vi "roboRIO v1.0 Read DIO.vi"(8 "error in (no error)":errorcluster, 10 "Channel List":T3, 11 "myRIO Ref In":T1) -> (0 "error out":errorcluster, 2 "bool Value List":bool[](array[boolean]), 3 "myRIO Ref Out":T1)   [LabVIEW 2021]
uses:
  <vilib>/myRIO/Common/Instrument Driver Framework/myRIO v1.0/DIO/typedefs/DIO Channels List.ctl
  <vilib>/myRIO/Common/Instrument Driver Framework/myRIO v1.0/DIO/typedefs/DIO Channels Enum.ctl
  <vilib>/myRIO/Common/Instrument Driver Framework/Utilities/typedefs/myRIO v1.0 Reference.ctl
  <vilib>/myRIO/Common/Instrument Driver Framework/Utilities/typedefs/Generic FPGA Reference.ctl
  <vilib>/myRIO/Common/Instrument Driver Framework/roboRIO v1.0/DIO/typedefs/roboRIO DIO FPGA Reference.ctl
  <vilib>/myRIO/Common/Instrument Driver Framework/roboRIO v1.0/DIO/typedefs/roboRIO DIO Bank Enum.ctl
  <vilib>/Utility/error.llb/Error Cluster From Error Code.vi
  <vilib>/rvi/errors/niLvFpgaAdjustHostInterfaceError.vi
  <vilib>/rvi/interface/nirviReadWriteControl/nirviReadWriteControl.xnode
  <vilib>/rvi/interface/Simulation/niFpgaSimulationCallBeginRW.vi
  NiFpgaLv.dll
panel:
  # "This VI reads boolean values from a list of user specified channels on\nthe myRIO v1.0 hardware. The value is read on the FPGA as a bit and \nconverted to a boolean. Please see Block Diagram for details."
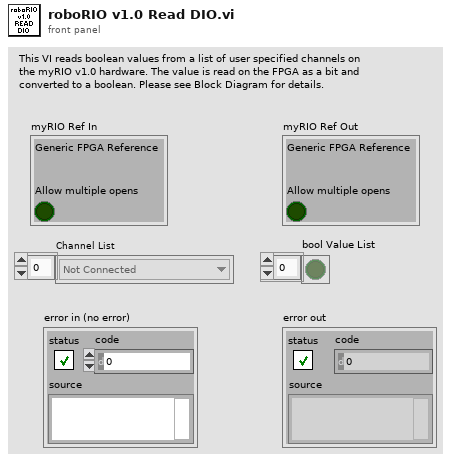
[diagram p1: front panel]
types:
  T1 = typedef "myRIO v1.0 Reference.ctl" = cluster{"Generic FPGA Reference":T2, "Allow multiple opens":bool}
  T2 = typedef "Generic FPGA Reference.ctl" = refnum<k20>
  T3 = typedef "DIO Channels List.ctl" = T4[]
  T4 = typedef "DIO Channels Enum.ctl" = enum16{"Not Connected", "C/DIO0", "C/DIO1", "C/DIO2", "C/DIO3", "C/DIO4", "C/DIO5", "C/DIO6", "C/DIO7", "A/DIO0", "A/DIO1", "A/DIO2", "A/DIO3", "A/DIO4", "A/DIO5", "A/DIO6", "A/DIO7", "A/DIO8", "A/DIO9", "A/DIO10", "A/DIO11", "A/DIO12", "A/DIO13", "A/DIO14", "A/DIO15", "A/DIO16", "A/DIO17", "A/DIO18", "A/DIO19", "B/DIO0", "B/DIO1", "B/DIO2", "B/DIO3", "B/DIO4", "B/DIO5", "B/DIO6", "B/DIO7", "B/DIO8", "B/DIO9", "B/DIO10", "B/DIO11", "B/DIO12", "B/DIO13", "B/DIO14", "B/DIO15", "B/DIO16", "B/DIO17", "B/DIO18", "B/DIO19", "LED0", "LED1", "LED2", "LED3", "Button0", "DIO/DIO0", "DIO/DIO1", "DIO/DIO2", "DIO/DIO3", "DIO/DIO4", "DIO/DIO5", "DIO/DIO6", "DIO/DIO7", "DIO/DIO8", "DIO/DIO9", "SPI/CS0", "SPI/CS1", "SPI/CS2", "SPI/CS3", "LED RADIO (Green)", "LED RADIO (Red)", "LED COMM (Green)", "LED COMM (Red)", "LED MODE (Green)", "LED MODE (Red)"}
  T5 = typedef "roboRIO DIO Bank Enum.ctl" = enum32{"None", "B/DIO7:0", "B/DIO15:8", "DIO/DIO7:0", "DIO/DIO9:8", "SPI/CS3:0", "LED", "Button0"}
  T6 = typedef "roboRIO DIO FPGA Reference.ctl" = refnum<k20>
  T7 = typedef "roboRIO DIO Bitmask to Channel Map.ctl" = cluster{"DIO Bank Enum":T5, "Bit":i32}
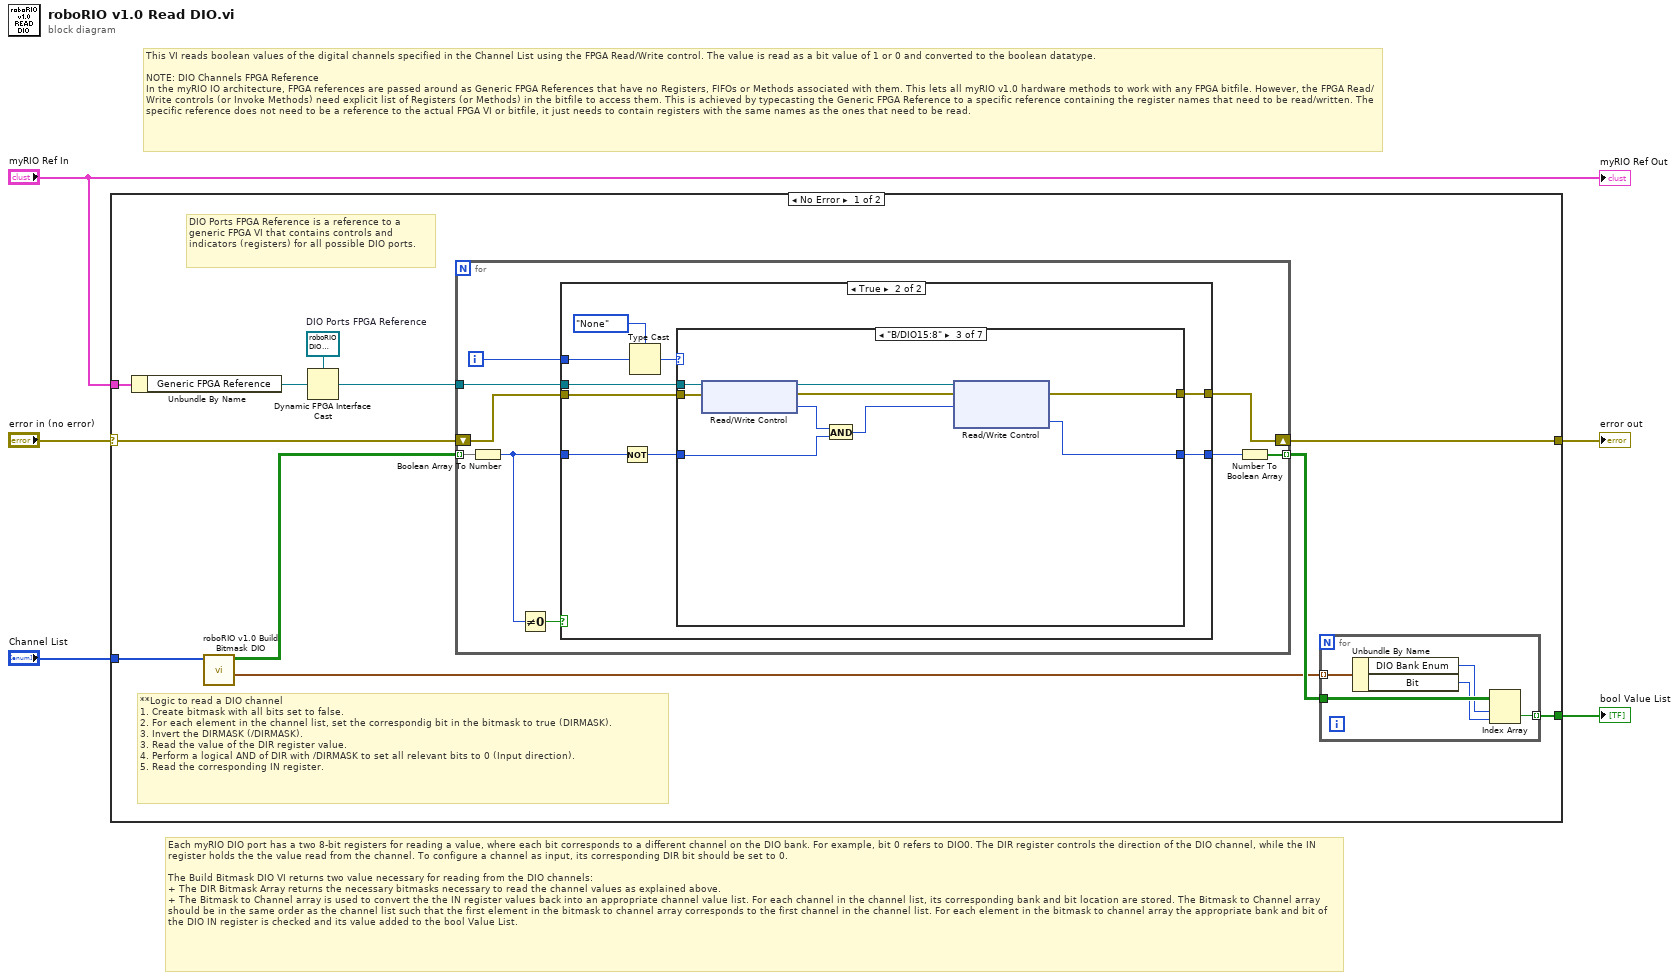
[diagram p0: block diagram]
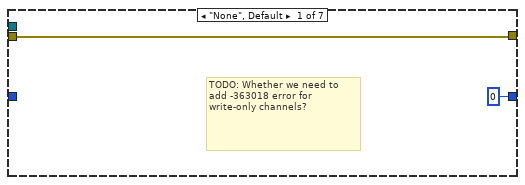
[diagram p3: hidden frame]
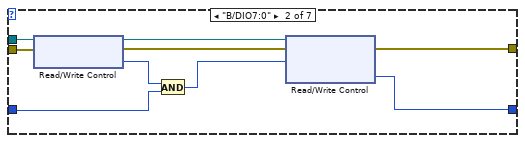
[diagram p4: hidden frame]
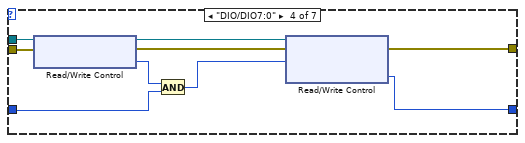
[diagram p5: hidden frame]
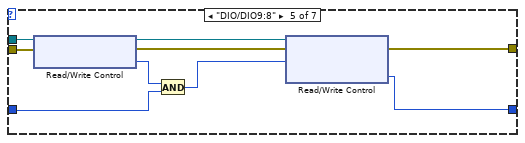
[diagram p6: hidden frame]
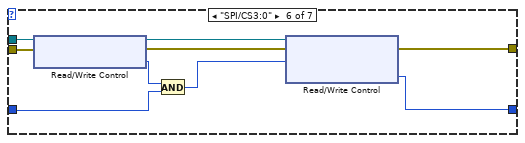
[diagram p7: hidden frame]
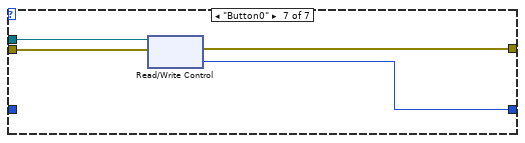
[diagram p8: hidden frame]
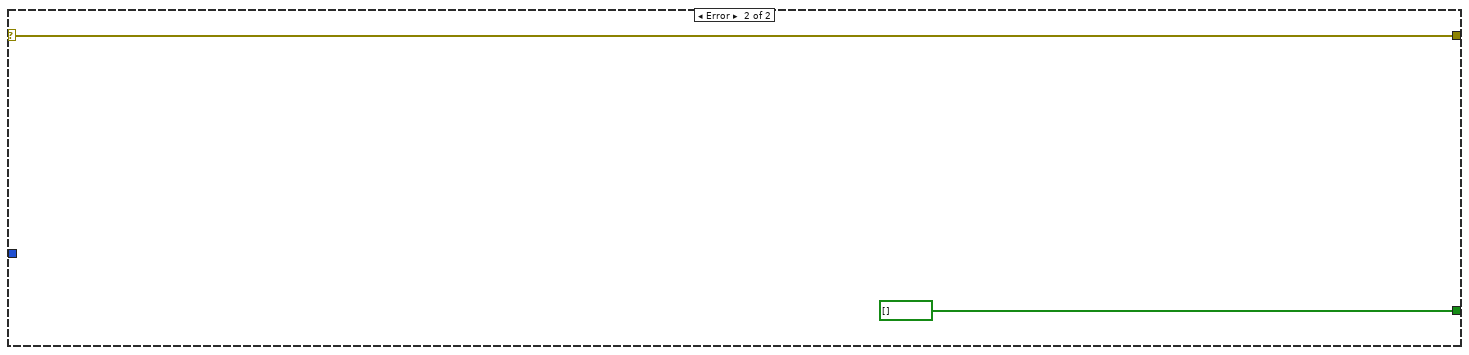
[diagram p9: hidden frame]
diagram:
  # "Each myRIO DIO port has a two 8-bit registers for reading a value, where each bit corresponds to a different channel on the DIO bank. For example, bit 0 refers to DIO0. The DIR register controls the direction of the DIO channel, while the IN register holds the the value read from the channel. To configure a channel as input, its corresponding DIR bit should be set to 0.\n\nThe Build Bitmask DIO VI returns two value necessary for reading from the DIO channels:\n+ The DIR Bitmask Array returns the necessary bitmasks necessary to read the channel values as explained above. \n+ The Bitmask to Channel array is used to convert the the IN register values back into an appropriate channel value list. For each channel in the channel list, its corresponding bank and bit location are stored. The Bitmask to Channel array should be in the same order as the channel list such that the first element in the bitmask to channel array corresponds to the first channel in the channel list. For each element in the bitmask to channel array the appropriate bank and bit of the DIO IN register is checked and its value added to the bool Value List."
  # "This VI reads boolean values of the digital channels specified in the Channel List using the FPGA Read/Write control. The value is read as a bit value of 1 or 0 and converted to the boolean datatype. \n\nNOTE: DIO Channels FPGA Reference\nIn the myRIO IO architecture, FPGA references are passed around as Generic FPGA References that have no Registers, FIFOs or Methods associated with them. This lets all myRIO v1.0 hardware methods to work with any FPGA bitfile. However, the FPGA Read/Write controls (or Invoke Methods) need explicit list of Registers (or Methods) in the bitfile to access them. This is achieved by typecasting the Generic FPGA Reference to a specific reference containing the register names that need to be read/written. The specific reference does not need to be a reference to the actual FPGA VI or bitfile, it just needs to contain registers with the same names as the ones that need to be read."
  n1 = case shown="No Error" "error in (no error)" {
    selector: "error in (no error)" -> [w7 w94]
    tunnel: "myRIO Ref In" -> [w13 _]
    tunnel: [w12 w94] -> w4
    tunnel: [w11 bool[] []] -> w2
    tunnel: "Channel List" -> [w10 _]
    frame No Error {
      w16 = T6 refnum  # DIO Ports FPGA Reference
      # "DIO Ports FPGA Reference is a reference to a generic FPGA VI that contains controls and indicators (registers) for all possible DIO ports."
      # "**Logic to read a DIO channel\n1. Create bitmask with all bits set to false.\n2. For each element in the channel list, set the correspondig bit in the bitmask to true (DIRMASK).\n3. Invert the DIRMASK (/DIRMASK).\n3. Read the value of the DIR register value.\n4. Perform a logical AND of DIR with /DIRMASK to set all relevant bits to 0 (Input direction).\n5. Read the corresponding IN register."
      n2 = Unbundle By Name(w13) -> ("Generic FPGA Reference"=w6:T2)
      n3 = call <vilib>:"roboRIO v1.0 Build Bitmask DIO.vi"("Channel List"=w10) -> ("Bitmask to Channel Array"=w8:T7[], "DIR Bitmask Array"=w9:bool[][])  [unwired: 8 in, 1 out]
      n4 = Dynamic FPGA Interface Cast(Session In=w16, Type=w6) -> (Session Out=w15:T6)
      n5 = for {
        tunnel: w9 -> [w28] mode=indexing
        tunnel: w15 -> [w30]
        shift-right: [w27] -> w12
        shift-left: w7 -> [w26]
        tunnel: [w24] -> w14 mode=indexing
        i -> [w29]
        n6 = Boolean Array To Number(Boolean array=w28) -> (number=w22:u8)
        n7 = Not Equal To 0?(x=w22) -> (x != 0?=w23:bool)
        n8 = case shown="True" w23 {
          tunnel: w30 -> [_ w41]
          tunnel: w29 -> [_ w40]
          tunnel: w22 -> [w31 w37]
          tunnel: [w32 w35] -> w27
          tunnel: w26 -> [w32 w34]
          tunnel: [w31 w33] -> w25
          frame False {
          }
          frame True {
            n9 = Not(x=w37) -> (.not. x?=w36:u8)
            n10 = Type Cast(type=roboRIO_DIO_Bank_Enum."None" ("DIO Bank Enum"), x=w40) -> (*(type *) &x=w38:T5)
            n11 = case shown="\"B/DIO15:8\"" w38 {
              tunnel: w41 -> [_ w52 w61 w70 w79 w88 w92]
              tunnel: w36 -> [_ w48 w57 w66 w75 w84 _]
              tunnel: [w43 w46 w55 w64 w73 w82 w91] -> w35
              tunnel: w34 -> [w43 w45 w54 w63 w72 w81 w90]
              tunnel: [u8 0 ("DIO.A_15:8.IN") w44 w53 w62 w71 w80 w89] -> w33
              frame "None", Default {
                # "TODO: Whether we need to add -363018 error for write-only channels?"
              }
              frame "B/DIO7:0" {
                n12 = xnode "Read/Write Control"("FPGA VI Reference In"=w52, "error in"=w45) -> ("FPGA VI Reference Out"=w51:T6, "error out"=w47:errorcluster, "DIO.B_7:0.DIR"=w50:u8)
                n13 = And(x=w50, y=w48) -> (x .and. y?=w49:u8)
                n14 = xnode "Read/Write Control"("FPGA VI Reference In"=w51, "error in"=w47, "DIO.B_7:0.DIR"=w49) -> ("error out"=w46:errorcluster, "DIO.B_7:0.IN"=w44:u8)  [unwired: 1 out]
              }
              frame "B/DIO15:8" {
                n15 = xnode "Read/Write Control"("FPGA VI Reference In"=w61, "error in"=w54) -> ("FPGA VI Reference Out"=w60:T6, "error out"=w56:errorcluster, "DIO.B_15:8.DIR"=w59:u8)
                n16 = And(x=w59, y=w57) -> (x .and. y?=w58:u8)
                n17 = xnode "Read/Write Control"("FPGA VI Reference In"=w60, "error in"=w56, "DIO.B_15:8.DIR"=w58) -> ("error out"=w55:errorcluster, "DIO.B_15:8.IN"=w53:u8)  [unwired: 1 out]
              }
              frame "DIO/DIO7:0" {
                n18 = xnode "Read/Write Control"("FPGA VI Reference In"=w70, "error in"=w63) -> ("FPGA VI Reference Out"=w69:T6, "error out"=w65:errorcluster, "DIO.DIO_7:0.DIR"=w68:u8)
                n19 = And(x=w68, y=w66) -> (x .and. y?=w67:u8)
                n20 = xnode "Read/Write Control"("FPGA VI Reference In"=w69, "error in"=w65, "DIO.DIO_7:0.DIR"=w67) -> ("error out"=w64:errorcluster, "DIO.DIO_7:0.IN"=w62:u8)  [unwired: 1 out]
              }
              frame "DIO/DIO9:8" {
                n21 = xnode "Read/Write Control"("FPGA VI Reference In"=w79, "error in"=w72) -> ("FPGA VI Reference Out"=w78:T6, "error out"=w74:errorcluster, "DIO.DIO_9:8.DIR"=w77:u8)
                n22 = And(x=w77, y=w75) -> (x .and. y?=w76:u8)
                n23 = xnode "Read/Write Control"("FPGA VI Reference In"=w78, "error in"=w74, "DIO.DIO_9:8.DIR"=w76) -> ("error out"=w73:errorcluster, "DIO.DIO_9:8.IN"=w71:u8)  [unwired: 1 out]
              }
              frame "SPI/CS3:0" {
                n24 = xnode "Read/Write Control"("FPGA VI Reference In"=w88, "error in"=w81) -> ("FPGA VI Reference Out"=w87:T6, "error out"=w83:errorcluster, "DIO.SPI_CS3:0.DIR"=w86:u8)
                n25 = And(x=w86, y=w84) -> (x .and. y?=w85:u8)
                n26 = xnode "Read/Write Control"("FPGA VI Reference In"=w87, "error in"=w83, "DIO.SPI_CS3:0.DIR"=w85) -> ("error out"=w82:errorcluster, "DIO.SPI_CS3:0.IN"=w80:u8)  [unwired: 1 out]
              }
              frame "Button0" {
                n27 = xnode "Read/Write Control"("FPGA VI Reference In"=w92, "error in"=w90) -> ("error out"=w91:errorcluster, "DI.BTN"=w89:u8)  [unwired: 1 out]
              }
            }
          }
        }
        n28 = Number To Boolean Array(number=w25) -> (Boolean array=w24:bool[])
      }
      n29 = for {
        tunnel: [w18] -> w11 mode=indexing
        tunnel: w14 -> [w21]
        tunnel: w8 -> [w17] mode=indexing
        n30 = Unbundle By Name(w17) -> ("DIO Bank Enum"=w20:T5, "Bit"=w19:i32)
        n31 = Index Array(array=w21, index (row)=w20, index (col)=w19) -> (element=w18:bool)
      }
    }
    frame Error {
    }
  }
  "error out" <- w4
  "bool Value List" <- w2
  "myRIO Ref Out" <- "myRIO Ref In"
